vi "macro_Pose3d_XYZ_Axis_AngleRad.vi"   [LabVIEW 2019, in "Trajectory_Library.lvlib"]
uses:
  Matrix_NormF.vi
  Quaternion_New.vi
  Rotation3d_Create_Default.vi
  <vilib>/Analysis/_algsub.llb/Matrix Norm.vi
  <vilib>/Analysis/_algsub.llb/Real Matrix Norm.vi
  Quaternion_New_Default.vi
  <vilib>/Analysis/Matrix/Numeric/Conversions/Array To Matrix.vi
  <vilib>/Analysis/Matrix/Numeric/Conversions/Array To Matrix - RA.vi
  Trajectory_Library.lvlib
types:
  T1 = typedef "Trajectory_Library.lvlib/ROTATION3D.ctl" = cluster{"Q_quaternion":T2}
  T2 = typedef "Trajectory_Library.lvlib/QUATERNION.ctl" = cluster{"R":dbl, "V":dbl[]}
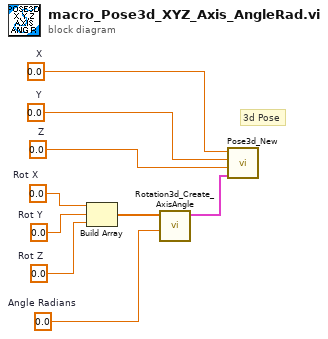
[diagram p0: block diagram]
diagram:
  w2 = 0.0  # X
  w3 = 0.0  # Y
  w4 = 0.0  # Z
  w6 = 0.0  # Rot Z
  w8 = 0.0  # Rot X
  w7 = 0.0  # Rot Y
  w1 = 0.0  # Angle Radians
  # "3d Pose"
  n1 = Build Array(w8, w7, w6) -> (w9:dbl[])
  n2 = call "Rotation3d_Create_AxisAngle.vi"("Angle"=w1, "Axis Vector"=w9) -> ("Rotation3d"=w5:T1)  [unwired: 9 in]
  n3 = call "Pose3d_New.vi"("Rotation3d"=w5, "z"=w4, "Y"=w3, "X"=w2) -> ()  [unwired: 7 in, 1 out]
